vi "VFP Network isStringProjectPath.vi"(5 "InitPath":string) -> (6 "isProjPath?":bool)   [LabVIEW 2016]
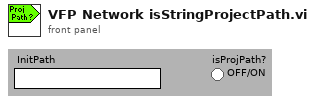
[diagram p1: front panel]
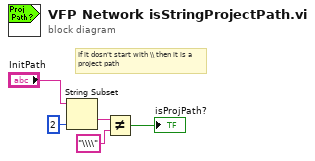
[diagram p0: block diagram]
diagram:
  # "If it dosn't start with \\\\ then it is a\nproject path"
  n1 = String Subset(string="InitPath", length (rest)=2 ("length (rest)")) -> (substring=w2:string)  [unwired: 1 in]
  n2 = Not Equal?(x=w2, y="\\\\") -> (x != y?=→"isProjPath?":bool)
